vi "Read DAQmx.AI.config.vi"(8 "error in (no error)":errorcluster, 11 "DAQmx.AI in":refnum<class "DAQmx.AI.lvclass">) -> (0 "error out":errorcluster, 2 "DAQmx.AI.Config":T1={"AI.Coupling"=10045, "input terminal configuration "=-1} {"input terminal configuration" items=["default"=-1, "RSE"=10083, "NRSE"=10078, "Differential"=10106, "Pseudodifferential"=12529]; "AI.Coupling" items=["AC"=10045, "DC"=10050, "GND"=10066]}, 3 "DAQmx.AI out":refnum<class "DAQmx.AI.lvclass">)   [LabVIEW 2016, in "DAQmx.AI.lvclass"]
uses:
  DAQmx.AI.lvclass
  Typedefs/DAQmx.AI.Config.ctl
  DAQmx.AI.lvclass/DAQmx.AI.ctl
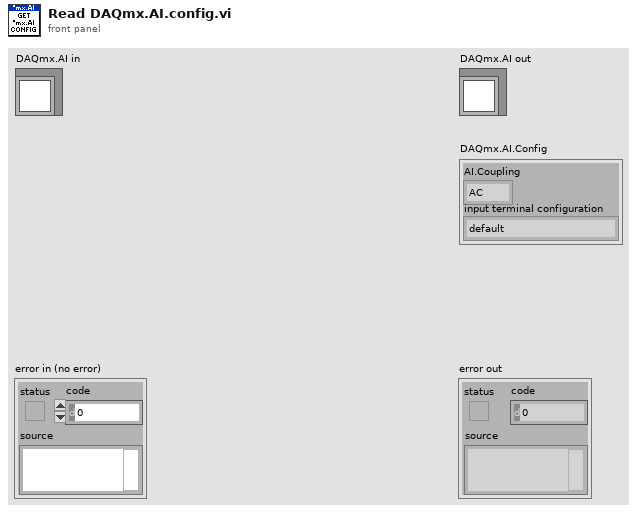
[diagram p1: front panel]
types:
  T1 = typedef "DAQmx.AI.lvclass/DAQmx.AI.Config.ctl" = cluster{"AI.Coupling":i32, "input terminal configuration ":i32}
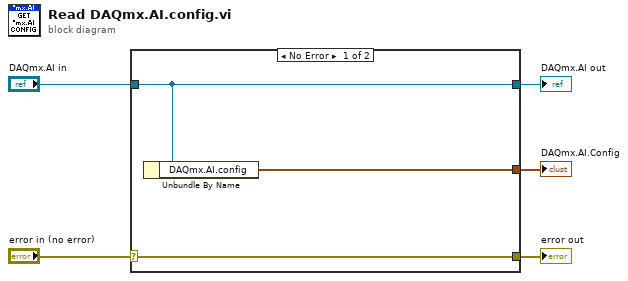
[diagram p0: block diagram]
diagram:
  n1 = case shown="No Error" "error in (no error)" {
    selector: "error in (no error)" -> [w8 w9]
    tunnel: [w8 w9] -> w4
    tunnel: [w7 w10] -> w2
    tunnel: "DAQmx.AI in" -> [w7 w10]
    tunnel: [w6 _] -> w1
    frame No Error {
      n2 = Unbundle By Name(w7) -> ("DAQmx.AI.config"=w6:T1)
    }
    frame Error {
    }
  }
  "error out" <- w4
  "DAQmx.AI out" <- w2
  "DAQmx.AI.Config" <- w1
